vi "Close Device.vi"(8 "Error In":errorcluster, 11 "LINX Device Config":T1) -> (0 "Error Out":errorcluster, 3 "LINX Device Config":T1)   [LabVIEW 2018, in "LVH-LINX.lvlib" / "Device.lvlib"]
doc: "Close the connection to the LINX device."
uses:
  Device.lvlib
  Type Defs/LINX Device Config.ctl
  Type Defs/Interface.ctl
  Type Defs/TCP Config.ctl
  Type Defs/Device Family.ctl
  LVH-LINX.lvlib
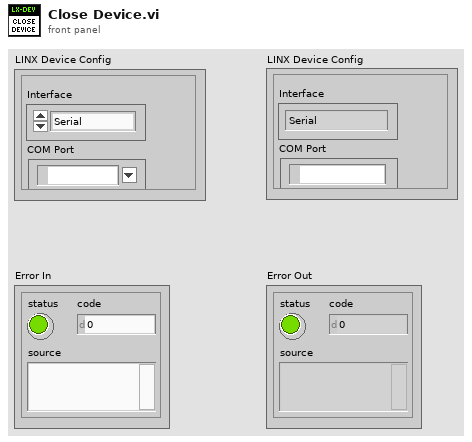
[diagram p1: front panel]
types:
  T1 = typedef "LVH-LINX.lvlib/Device.lvlib/LINX Device Config.ctl" = cluster{"Interface":T2, "COM Port":refnum<visa-resource-name>, "TCP Configuration":T3, "Device Family":T4, "Device ID":u8, "Device Name":string, "TCP Ref":refnum<k5>}
  T2 = typedef "LVH-LINX.lvlib/Interface.ctl" = enum16{"Serial", "TCP"}
  T3 = typedef "LVH-LINX.lvlib/Device.lvlib/TCP Config.ctl" = cluster{"IP Address":string, "Port":u16}
  T4 = typedef "LVH-LINX.lvlib/Device Family.ctl" = enum8{"National Instruments", "Digilent", "Arduino"}
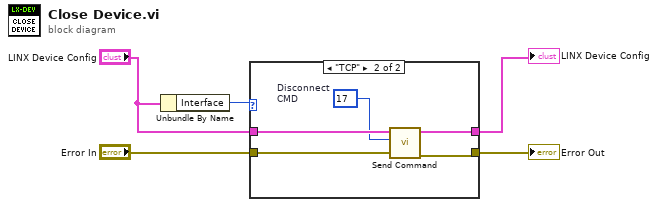
[diagram p0: block diagram]
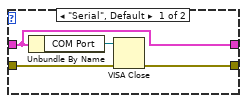
[diagram p2: hidden frame]
diagram:
  n1 = Unbundle By Name("LINX Device Config") -> ("Interface"=w3:T2)
  n2 = case shown="\"TCP\"" w3 {
    tunnel: "LINX Device Config" -> [w6 w12]
    tunnel: "Error In" -> [w8 w11]
    tunnel: [w7 w14] -> w4
    tunnel: [w6 w13] -> w1
    frame "Serial", Default {
      n3 = Unbundle By Name(w6) -> ("COM Port"=w9:refnum<visa-resource-name>)
      n4 = VISA Close(VISA resource name=w9, error in (no error)=w8) -> (error out=w7:errorcluster)
    }
    frame "TCP" {
      w10 = u16 17  # Disconnect CMD
      n5 = call "Send Command.vi"("Error In"=w11, "CMD"=w10, "LINX Device Config"=w12) -> ("Error Out"=w14:errorcluster, "LINX Device Config"=w13:T1)  [unwired: 5 in, 2 out]
    }
  }
  "Error Out" <- w4
  "LINX Device Config" <- w1
